vi "StartTimesSratchpad.vi"() -> ()   [LabVIEW 2013]
panel:
  out "Start Times":i32[][](array[numeric])
  in  "Completion Times":i32[][](array[numeric])
  in  "Brucker j4-per0-1 Processing Times(MxJ)":i32[][](array[numeric])=[[1, 62, 270, 667], [303, 255, 170, 272], [66, 556, 373, 5], [630, 127, 187, 56]]
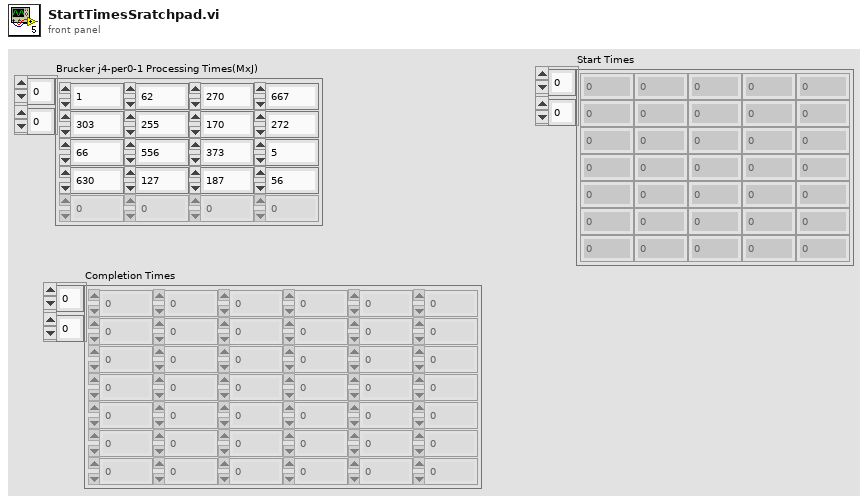
[diagram p1: front panel]
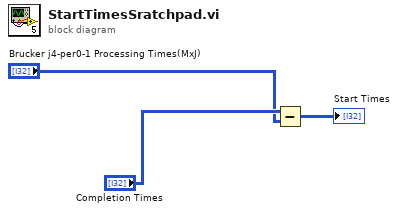
[diagram p0: block diagram]
diagram:
  n1 = Subtract(x="Completion Times", y="Brucker j4-per0-1 Processing Times(MxJ)") -> (x-y=→"Start Times":i32[][])
